vi "Flatten UIP Value.vi"(11 "UIP In":refnum<class "TemplateUIP.lvclass">) -> (0 "Error Out":errorcluster, 2 "String Value":string, 3 "UIP Out":refnum<class "TemplateUIP.lvclass">)   [LabVIEW 2015, in "TemplateUIP.lvclass"]
uses:
  TemplateUIP.lvclass
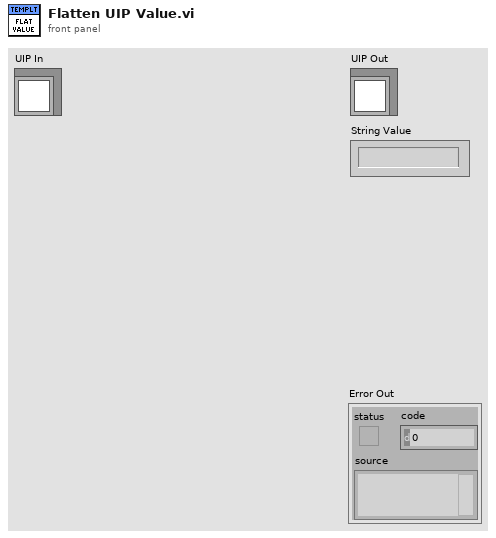
[diagram p1: front panel]
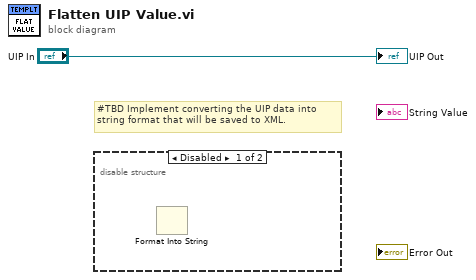
[diagram p0: block diagram]
diagram:
  # "#TBD Implement converting the UIP data into\nstring format that will be saved to XML."
  n1 = disable-structure shown="Disabled" {
    frame Disabled {
      n2 = Format Into String "Format Into String"() -> ()  [unwired: 4 in, 2 out]
    }
    frame Enabled {
    }
  }
  "UIP Out" <- "UIP In"
